vi "Semaphores.vi"() -> ()   [LabVIEW 2019]
uses:
  <vilib>/measure/NI_MABase.lvlib
panel:
  out "String":string
  out "LED-3":bool
  out "LED-2":bool
  out "LED-1":bool
  out "L-3":waveform(dbl)(graph)={"t0"=timestamp(206.0 s since 1904-01-01), "dt"=0.001, "Y"=array[1000 elements]} caption="L-2"
  out "L-2":waveform(dbl)(graph)={"t0"=timestamp(119.0 s since 1904-01-01), "dt"=0.001, "Y"=array[1000 elements]}
  out "L-1":waveform(dbl)(graph)={"t0"=timestamp(86.0 s since 1904-01-01), "dt"=0.001, "Y"=array[1000 elements]}
  in  "?":bool
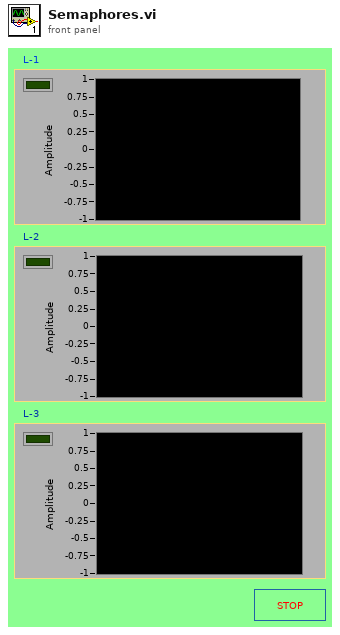
[diagram p1: front panel]
types:
  T1 = typedef "Semaphore RefNum" = refnum<k1>
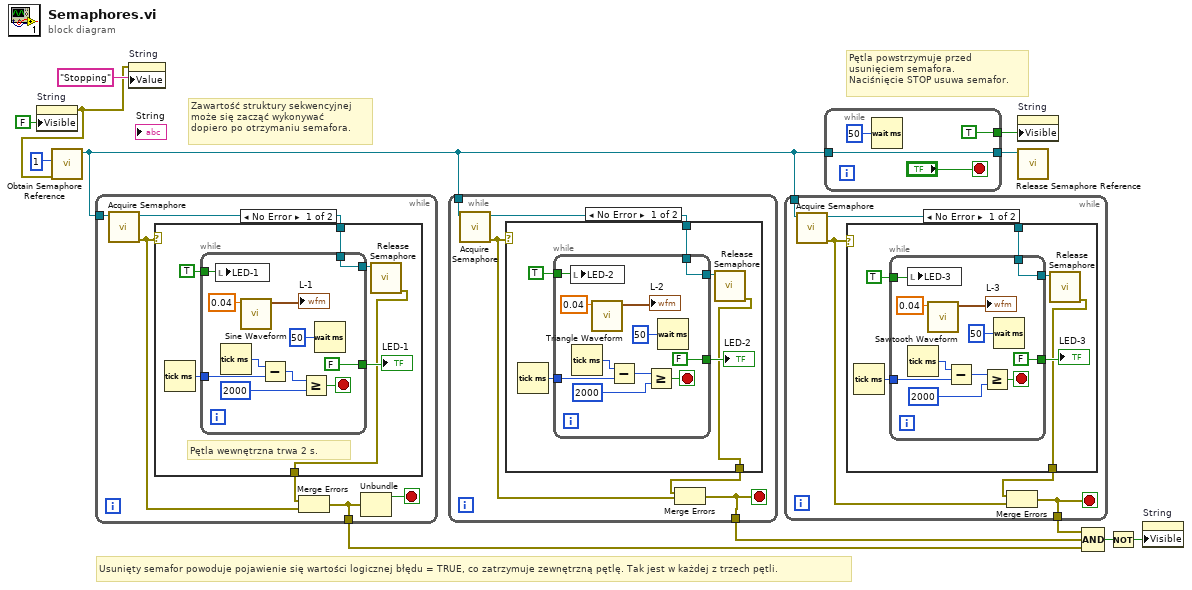
[diagram p0: block diagram]
diagram:
  # "Zawartość struktury sekwencyjnej \nmoże się zacząć wykonywać \ndopiero po otrzymaniu semafora."
  # "Usunięty semafor powoduje pojawienie się wartości logicznej błędu = TRUE, co zatrzymuje zewnętrzną pętlę. Tak jest w każdej z trzech pętli."
  # "Pętla powstrzymuje przed\nusunięciem semafora. \nNaciśnięcie STOP usuwa semafor."
  n1 = property on="String" class="Str"("Visible"=FALSE) -> (error out=w1:errorcluster)  [unwired: 2 in, 1 out]
  n2 = call <vilib>:"Obtain Semaphore Reference.vi"("error in (no error)"=w1, "size (1)"=1) -> ("semaphore"=w10:T1)  [unwired: 3 in, 2 out]
  n3 = while {
    tunnel: w10 -> [w17]
    tunnel: [w13] -> w3
    stop <- w16 stop-if-true
    n4 = call <vilib>:"Acquire Semaphore.vi"("semaphore"=w17) -> ("error out"=w15:errorcluster, "semaphore out"=w18:T1)  [unwired: 4 in, 1 out]
    n5 = case shown="No Error" w15 {
      tunnel: w18 -> [w24 _]
      tunnel: [w19 _] -> w14
      frame No Error {
        # "Pętla wewnętrzna trwa 2 s."
        n6 = Tick Count (ms)() -> (millisecond timer value=w23:u32)
        n7 = while {
          tunnel: w23 -> [w32]
          tunnel: w24 -> [w29]
          tunnel: [w29] -> w22
          tunnel: [FALSE] -> w21
          tunnel: TRUE ("LED-1") -> [w25]
          stop <- w30 stop-if-true
          n8 = local write "LED-1"(w25) -> ()
          n9 = Tick Count (ms)() -> (millisecond timer value=w33:u32)
          n10 = call <vilib>:"Sine Waveform.vi"("frequency"=0.04) -> ("signal out"=→"L-1":waveform(dbl))  [unwired: 9 in, 1 out]
          n11 = Subtract(x=w33, y=w32) -> (x-y=w27:u32)
          n12 = Greater Or Equal?(x=w27, y=u32 2000) -> (x >= y?=w30:bool)
          n13 = Wait (ms)(milliseconds to wait=u32 50) -> ()  [unwired: 1 out]
        }
        "LED-1" <- w21
        n14 = call <vilib>:"Release Semaphore.vi"("semaphore"=w22) -> ("error out"=w19:errorcluster)  [unwired: 5 in, 1 out]
      }
      frame Error {
      }
    }
    n15 = Merge Errors(w14, w15) -> (w13:errorcluster)
    n16 = Unbundle(w13) -> ("status"=w16:bool)  [unwired: 2 out]
  }
  n17 = property on="String" class="Str"(error in=w1, "Value"="Stopping" ("String")) -> ()  [unwired: 1 in, 2 out]
  n18 = while {
    tunnel: w10 -> [w39]
    tunnel: [w38] -> w6
    stop <- w38 stop-if-true
    n19 = call <vilib>:"Acquire Semaphore.vi"("semaphore"=w39) -> ("error out"=w37:errorcluster, "semaphore out"=w40:T1)  [unwired: 4 in, 1 out]
    n20 = case shown="No Error" w37 {
      tunnel: w40 -> [w46 _]
      tunnel: [w41 _] -> w36
      frame No Error {
        n21 = Tick Count (ms)() -> (millisecond timer value=w45:u32)
        n22 = while {
          tunnel: w45 -> [w54]
          tunnel: w46 -> [w51]
          tunnel: [w51] -> w44
          tunnel: [FALSE] -> w43
          tunnel: TRUE ("LED-2") -> [w47]
          stop <- w52 stop-if-true
          n23 = local write "LED-2"(w47) -> ()
          n24 = Tick Count (ms)() -> (millisecond timer value=w55:u32)
          n25 = call <vilib>:"Triangle Waveform.vi"("frequency"=0.04) -> ("signal out"=→"L-2":waveform(dbl))  [unwired: 9 in, 1 out]
          n26 = Subtract(x=w55, y=w54) -> (x-y=w49:u32)
          n27 = Greater Or Equal?(x=w49, y=u32 2000) -> (x >= y?=w52:bool)
          n28 = Wait (ms)(milliseconds to wait=u32 50) -> ()  [unwired: 1 out]
        }
        "LED-2" <- w43
        n29 = call <vilib>:"Release Semaphore.vi"("semaphore"=w44) -> ("error out"=w41:errorcluster)  [unwired: 5 in, 1 out]
      }
      frame Error {
      }
    }
    n30 = Merge Errors(w36, w37) -> (w38:errorcluster)
  }
  n31 = while {
    tunnel: w10 -> [w61]
    tunnel: [w59] -> w7
    stop <- w59 stop-if-true
    n32 = call <vilib>:"Acquire Semaphore.vi"("semaphore"=w61) -> ("error out"=w60:errorcluster, "semaphore out"=w62:T1)  [unwired: 4 in, 1 out]
    n33 = case shown="No Error" w60 {
      tunnel: w62 -> [w68 _]
      tunnel: [w63 _] -> w58
      frame No Error {
        n34 = Tick Count (ms)() -> (millisecond timer value=w67:u32)
        n35 = while {
          tunnel: w67 -> [w76]
          tunnel: w68 -> [w73]
          tunnel: [w73] -> w66
          tunnel: [FALSE] -> w65
          tunnel: TRUE ("LED-3") -> [w69]
          stop <- w74 stop-if-true
          n36 = local write "LED-3"(w69) -> ()
          n37 = Tick Count (ms)() -> (millisecond timer value=w77:u32)
          n38 = call <vilib>:"Sawtooth Waveform.vi"("frequency"=0.04) -> ("signal out"=→"L-3":waveform(dbl))  [unwired: 9 in, 1 out]
          n39 = Subtract(x=w77, y=w76) -> (x-y=w71:u32)
          n40 = Greater Or Equal?(x=w71, y=u32 2000) -> (x >= y?=w74:bool)
          n41 = Wait (ms)(milliseconds to wait=u32 50) -> ()  [unwired: 1 out]
        }
        "LED-3" <- w65
        n42 = call <vilib>:"Release Semaphore.vi"("semaphore"=w66) -> ("error out"=w63:errorcluster)  [unwired: 5 in, 1 out]
      }
      frame Error {
      }
    }
    n43 = Merge Errors(w58, w60) -> (w59:errorcluster)
  }
  n44 = while {
    tunnel: w10 -> [w83]
    tunnel: [w83] -> w11
    tunnel: [TRUE] -> w8
    stop <- "?" stop-if-true
    n45 = Wait (ms)(milliseconds to wait=u32 50) -> ()  [unwired: 1 out]
  }
  n46 = property on="String" class="Str"("Visible"=w8) -> ()  [unwired: 2 in, 2 out]
  n47 = call <vilib>:"Release Semaphore Reference.vi"("semaphore"=w11) -> ()  [unwired: 9 in, 2 out]
  n48 = Compound Arithmetic op=AND(w7, w6, w3) -> (w5:bool)
  n49 = Not(x=w5) -> (.not. x?=w4:bool)
  n50 = property on="String" class="Str"("Visible"=w4) -> ()  [unwired: 2 in, 2 out]
